vi "Add To DAQmx Task.vi"(6 "Ignore Cal? (F)":bool, 7 "Strain in":refnum<class "Strain.lvclass">, 8 "error in (no error)":errorcluster, 9 "Scale Name":string, 10 "Chassis Name":string, 11 "task in":refnum<k21>) -> (0 "error out":errorcluster, 2 "Phys Chan Added":string, 3 "task out":refnum<k21>)   [LabVIEW 2012, in "Measurement Channels.lvlib" / "Strain.lvclass"]
uses:
  Strain.lvclass
  Strain.lvclass/Strain.ctl
  Class Channel/Read ChanName.vi
  Class Channel/Read Alias.vi
  <vilib>/DAQmx/create/scale.llb/DAQmx Create Scale (Linear).vi
  <vilib>/DAQmx/create/channels.llb/DAQmx Create Channel (AI-Strain-Strain Gage).vi
  <resource>/objmgr/daqmx.rc
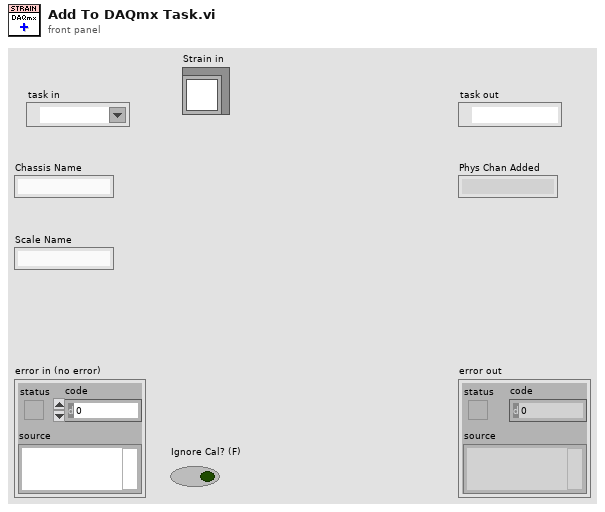
[diagram p1: front panel]
types:
  T1 = cluster{"gage factor":dbl, "nominal gage resistance":dbl, "poisson ratio":dbl}
  T2 = cluster{"strain configuration":i32, "lead wire resistance":dbl, "initial bridge voltage":dbl, "voltage excitation source":i32, "voltage excitation value":dbl}
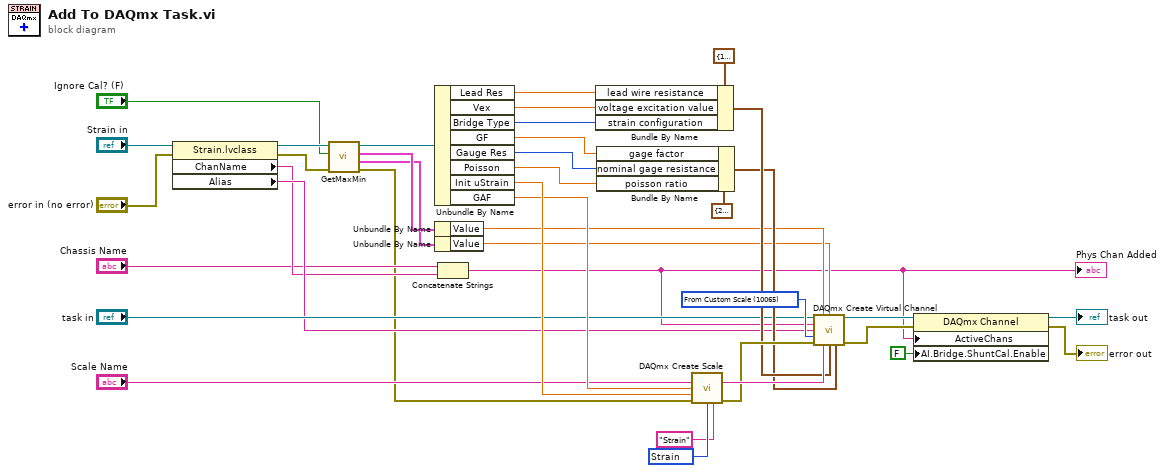
[diagram p0: block diagram]
diagram:
  w34 = 10065 items=["Strain"=10299, "From Custom Scale"=10065] ("units")
  w30 = 10299 items=["Volts"=10348, "Amps"=10342, "Deg F"=10144, "Deg C"=10143, "Deg R"=10145, "Kelvins"=10325, "Strain"=10299, "Ohms"=10384, "Hz"=10373, "Seconds"=10364, "Meters"=10219, "Inches"=10379, "Degrees"=10146, "Radians"=10273, "g"=10186, "m/s^2"=12470, "Pascals"=10081, "Newtons"=15875, "Pounds"=15876, "kgf"=15877, "psi"=15879, "bar"=15880, "Nm"=15881, "oz-in"=15882, "lb-in"=15883, "lb-ft"=15884, "Volts/Volt"=15896, "mVolts/Volt"=15897, "From TEDS"=12516] ("pre-scaled units")
  n1 = property class="Strain.lvclass"(reference="Strain in", error in="error in (no error)") -> (reference out=w12:refnum<class "Strain.lvclass">, error out=w4:errorcluster, "ChanName"=w8:string, "Alias"=w9:string)
  n2 = call-dynamic "GetMaxMin.vi"("error in (no error)"=w4, "Ignore Cal? (F)"="Ignore Cal? (F)", "Strain in"=w12) -> ("error out"=w3:errorcluster, "Min"=w17:cluster{"Value":dbl, "Text":string}, "Max"=w18:cluster{"Value":dbl, "Text":string}, "Strain out"=w19:refnum<class "Strain.lvclass">)  [unwired: 5 in]
  n3 = Unbundle By Name(w19) -> ("Lead Res"=w35:dbl, "Vex"=w22:dbl, "Bridge Type"=w23:u16, "GF"=w26:dbl, "Gauge Res"=w27:i32, "Poisson"=w28:dbl, "Init uStrain"=w36:dbl, "GAF"=w32:dbl)
  n4 = Unbundle By Name(w18) -> ("Value"=w16:dbl)
  n5 = Unbundle By Name(w17) -> ("Value"=w15:dbl)
  n6 = Concatenate Strings("Chassis Name", w8) -> (w2:string)
  "Phys Chan Added" <- w2
  n7 = Bundle By Name(cluster=T2 {"strain configuration"=10183, "lead wire resistance"=0.0, "initial bridge voltage"=0.0, "voltage excitation source"=10200, "voltage excitation value"=2.5} ("bridge information"), "lead wire resistance"=w35, "voltage excitation value"=w22, "strain configuration"=w23) -> (w25:T2)
  n8 = Bundle By Name(cluster=T1 {"gage factor"=2.0, "nominal gage resistance"=350.0, "poisson ratio"=0.3} ("strain gage information"), "gage factor"=w26, "nominal gage resistance"=w27, "poisson ratio"=w28) -> (w24:T1)
  n9 = call-poly <vilib>:"DAQmx Create Scale.vi"("name"="Scale Name", "slope"=w32, "y-intercept"=w36, "error in"=w3, "pre-scaled units"=w30, "scaled units"="Strain") -> ("scale out"=w33:tag, "error out"=w31:errorcluster)  [unwired: 8 in]
  n10 = call-poly <vilib>:"DAQmx Create Virtual Channel.vi"("task in"="task in", "maximum value"=w16, "minimum value"=w15, "physical channels"=w2, "name to assign"=w9, "units"=w34, "error in"=w31, "custom scale name"=w33, "bridge information"=w25, "strain gage information"=w24) -> ("task out"=w37:refnum<k21>, "error out"=w38:errorcluster)  [unwired: 4 in]
  n11 = property class="DAQmx Channel"(reference=w37, error in=w38, "ActiveChans"=w2, "AI.Bridge.ShuntCal.Enable"=FALSE) -> (reference out=→"task out":refnum<k21>, error out=→"error out":errorcluster)
